vi "Test subvi.vi"() -> ()   [LabVIEW 2021]
panel:
  out "error out 2":errorcluster
  out "error out":errorcluster
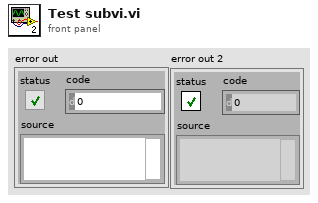
[diagram p1: front panel]
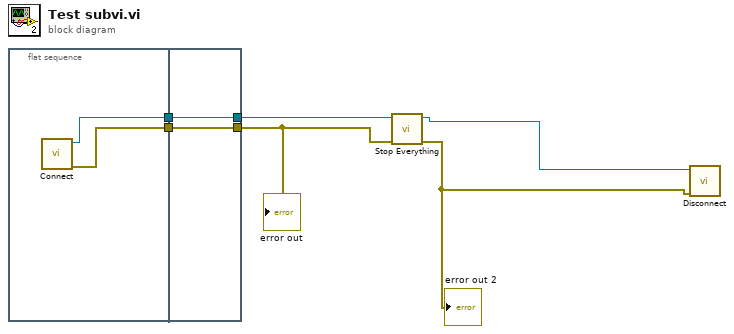
[diagram p0: block diagram]
diagram:
  n1 = flat-sequence {
    tunnel: [w8] -> w4
    tunnel: [w7] -> w3
    tunnel: [w9] -> w5
    tunnel: [w10] -> w6
    tunnel: w4 -> [w10]
    tunnel: w3 -> [w9]
    frame #0 {
      n2 = call "Connect.vi"() -> ("TCP slave instance"=w8:refnum<class "Modbus Slave.lvclass">, "error out"=w7:errorcluster)  [unwired: 8 in]
    }
    frame #1 {
    }
  }
  n3 = call "Stop Everything.vi"("error in"=w5, "TCP slave instance"=w6) -> ("error out"=w1:errorcluster, "TCP slave instance"=w2:refnum<class "Modbus Slave.lvclass">)  [unwired: 8 in]
  "error out 2" <- w1
  n4 = call "Disconnect.vi"("error in (no error)"=w1, "TCP slave instance"=w2) -> ()  [unwired: 10 in]
  "error out" <- w5
